vi "Cmd_UpdatePositions.vi"(11 "Msg Data":variant) -> (2 "Magnet Z":dbl, 3 "Numeric":dbl)   [LabVIEW 2011]
uses:
  Main/GlobalVariables.vi
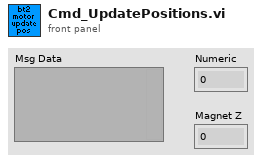
[diagram p1: front panel]
types:
  T1 = typedef "MotorPosType.ctl" = cluster{"Magnet Z":dbl, "Magnet rotation":dbl, "Camera":T2, "Piezo XY":T2, "Piezo Z":dbl}
  T2 = typedef "XYf.ctl" = cluster{"X":sgl, "Y":sgl}
  T3 = typedef "MotorConfigType.ctl" = cluster{"Offset":T1, "Maximum pos":T1, "Min limited?":T4, "Max limited?":T4, "Has velocity support":T4, "Default velocity":T1}
  T4 = typedef "MotorPosFlagsType.ctl" = cluster{"Magnet Z":bool, "Magnet rotation":bool, "Camera":cluster{"X":bool, "Y":bool}, "Piezo XY":cluster{"X":bool, "Y":bool}, "Piezo Z":bool}
  T5 = typedef "MotorStateType.ctl" = cluster{"Enabled?":bool, "Current Position":T1, "Update counter":i32}
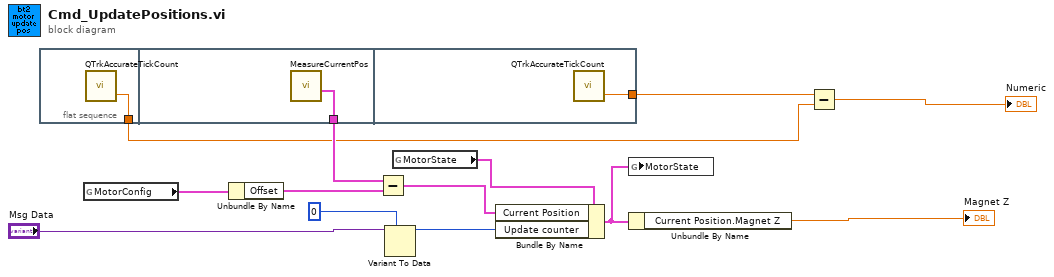
[diagram p0: block diagram]
diagram:
  n1 = flat-sequence {
    tunnel: [w14] -> w3
    tunnel: [w15] -> w7
    tunnel: [w16] -> w2
    frame #0 {
      n2 = call "QTrkAccurateTickCount.vi"() -> ("seconds"=w14:dbl)  [unwired: 2 in, 1 out]
    }
    frame #1 {
      n3 = call "MeasureCurrentPos.vi"() -> ("Current Position"=w15:T1)  [unwired: 11 in]
    }
    frame #2 {
      n4 = call "QTrkAccurateTickCount.vi"() -> ("seconds"=w16:dbl)  [unwired: 2 in, 1 out]
    }
  }
  n5 = global read "GlobalVariables.vi" "MotorConfig"() -> (w5:T3)
  n6 = Unbundle By Name(w5) -> ("Offset"=w6:T1)
  n7 = Subtract(x=w7, y=w6) -> (x-y=w8:T1)
  n8 = Variant To Data(type=0 ("Update counter"), Variant="Msg Data") -> (data=w11:i32)  [unwired: 1 in, 1 out]
  n9 = global read "GlobalVariables.vi" "MotorState"() -> (w1:T5)
  n10 = Bundle By Name(cluster=w1, "Current Position"=w8, "Update counter"=w11) -> (w12:T5)
  n11 = global write "GlobalVariables.vi" "MotorState"(w12) -> ()
  n12 = Unbundle By Name(w12) -> ("Current Position.Magnet Z"=→"Magnet Z":dbl)
  n13 = Subtract(x=w2, y=w3) -> (x-y=→"Numeric":dbl)
